vi "Memory.Pointer.New.vi"(8 "error in (no error)":errorcluster, 11 "size":u64 format="%08x bytes") -> (0 "error out":errorcluster, 3 "pointer":refnum<class "Memory.Pointer.lvclass">)   [LabVIEW 2016, in "Memory Manager.lvlib" / "Memory.Pointer.lvclass"]
uses:
  Memory.Pointer.lvclass
  Memory.Pointer.lvclass/Memory.Pointer.ctl
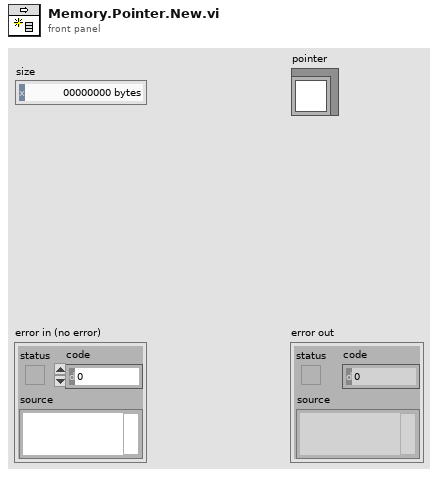
[diagram p1: front panel]
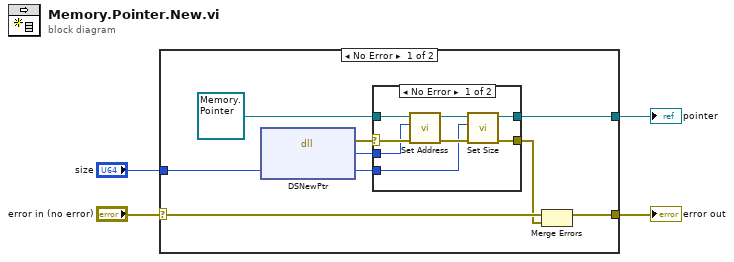
[diagram p0: block diagram]
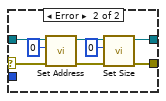
[diagram p2: hidden frame]
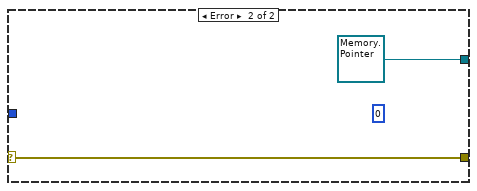
[diagram p3: hidden frame]
diagram:
  n1 = case shown="No Error" "error in (no error)" {
    selector: "error in (no error)" -> [w11 w31]
    tunnel: [w13 w31] -> w4
    tunnel: [w5 refnum<class "Memory.Pointer.lvclass"> refnum ("Pointer out")] -> w3
    tunnel: "size" -> [w6 _]
    frame No Error {
      n2 = dll-call lib="LabVIEW" fn="DSNewPtr"("size"=w6) -> (error out=w8:errorcluster, "pointer"=w10:u64, "size"=w9:u64)  [unwired: 3 in, 1 out]
      n3 = case shown="No Error" w8 {
        selector: w8 -> [w20 w28]
        tunnel: refnum<class "Memory.Pointer.lvclass"> refnum ("Pointer") -> [w21 w29]
        tunnel: w10 -> [w19 _]
        tunnel: [w16 w25] -> w5
        tunnel: w9 -> [w14 _]
        tunnel: [w15 w24] -> w7
        frame No Error {
          n4 = call "Set Address.vi"("error in (no error)"=w20, "address"=w19, "Pointer in"=w21) -> ("error out"=w17:errorcluster, "Pointer out"=w18:refnum<class "Memory.Pointer.lvclass">)  [unwired: 7 in]
          n5 = call "Set Size.vi"("error in (no error)"=w17, "size"=w14, "Pointer in"=w18) -> ("error out"=w15:errorcluster, "Pointer out"=w16:refnum<class "Memory.Pointer.lvclass">)  [unwired: 7 in]
        }
        frame Error {
          n6 = call "Set Address.vi"("error in (no error)"=w28, "address"=u64 0, "Pointer in"=w29) -> ("error out"=w26:errorcluster, "Pointer out"=w27:refnum<class "Memory.Pointer.lvclass">)  [unwired: 7 in]
          n7 = call "Set Size.vi"("error in (no error)"=w26, "size"=u64 0, "Pointer in"=w27) -> ("error out"=w24:errorcluster, "Pointer out"=w25:refnum<class "Memory.Pointer.lvclass">)  [unwired: 7 in]
        }
      }
      n8 = Merge Errors(w11, w7) -> (w13:errorcluster)
    }
    frame Error {
      (unwired) u64 0 ("size")
    }
  }
  "error out" <- w4
  "pointer" <- w3
